vi "Reprint_Data.vi"(11 "recordset data":variant[][](array[variant])) -> (0 "error out":errorcluster, 1 "Status":string, 2 "Pass Date":timestamp, 3 "Serail No":i32, 4 "RFID":string, 6 "reversed":string)   [LabVIEW 2020]
uses:
  <vilib>/addons/database/_DB Variant To Data/Database Variant To Data.xnode
panel:
  out "Barcode":string
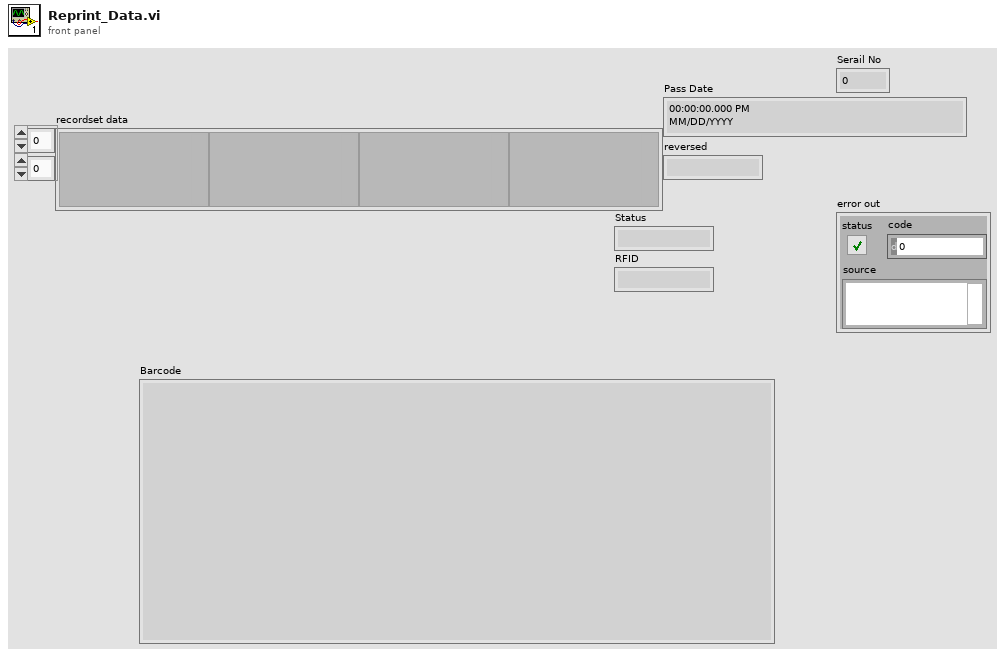
[diagram p1: front panel]
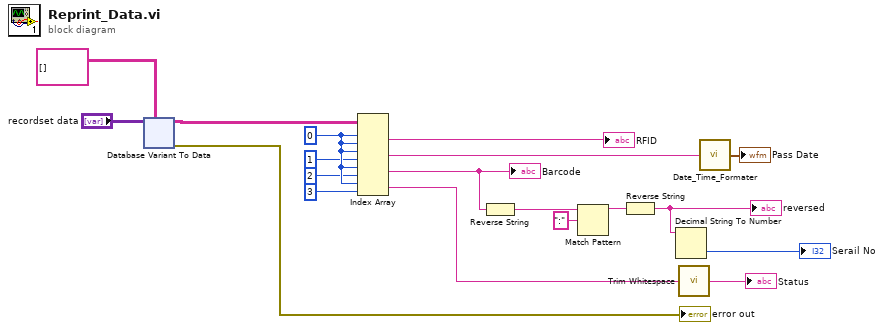
[diagram p0: block diagram]
diagram:
  w19 = 0 ("index (row)")
  n1 = xnode "Database Variant To Data"("database variant"="recordset data", "type"=string[][] []) -> ("data"=w13:string[][], "error out"=→"error out":errorcluster)  [unwired: 1 in]
  n2 = Index Array(array=w13, index (row) #1=w19, index (col) #1=w19, index (row) #2=w19, index (col) #2=1 ("disabled index (col)"), index (row) #3=w19, index (col) #3=2 ("disabled index (col)"), index (row) #4=w19, index (col) #4=3 ("disabled index (col)")) -> (element #1=→"RFID":string, element #2=w12:string, element #3=w10:string, element #4=w4:string)
  "Barcode" <- w10
  n3 = Reverse String(1:w10) -> (0:w9:string)
  n4 = Match Pattern(string=w9, regular expression=":") -> (before substring=w7:string)  [unwired: 1 in, 3 out]
  n5 = Reverse String(1:w7) -> (0:w1:string)
  "reversed" <- w1
  n6 = Decimal String To Number(string=w1) -> (number=→"Serail No":i32)  [unwired: 2 in, 1 out]
  n7 = call <vilib>:"Trim Whitespace.vi"("string"=w4) -> ("trimmed string"=→"Status":string)  [unwired: 1 in]
  n8 = call "Date_Time_Formater.vi"("Date In"=w12) -> ("Date Out"=→"Pass Date":timestamp)
